vi "Tap Handler.vi"(8 "error in (no error)":errorcluster) -> (0 "error out":errorcluster)   [LabVIEW 2014]
uses:
  STD - Tap Mode.ctl
  Globals.vi
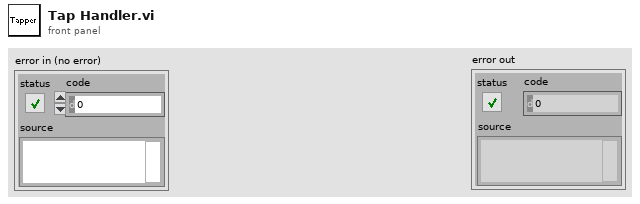
[diagram p1: front panel]
types:
  T1 = typedef "STD - Tap Mode.ctl" = enum32{"No Action", "Stay Level", "Rise", "Fall", "Calibrate"}
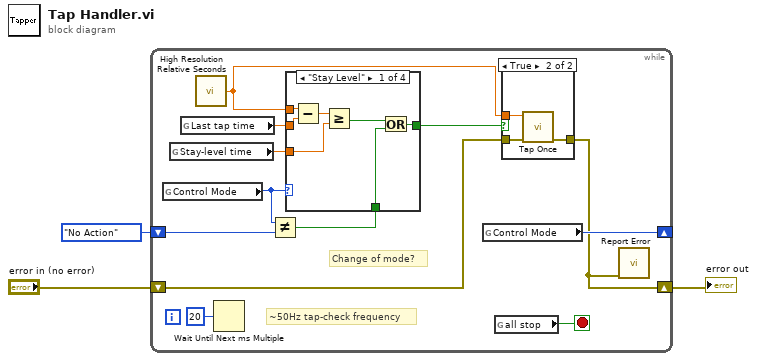
[diagram p0: block diagram]
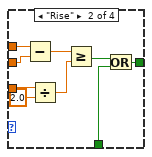
[diagram p2: hidden frame]
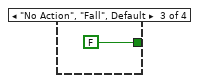
[diagram p3: hidden frame]
diagram:
  n1 = while {
    shift-right: [w11] -> _
    shift-left: STD_-_Tap_Mode."No Action" ("Control Mode") -> [w10]
    shift-right: [w4] -> w2
    shift-left: "error in (no error)" -> [w6]
    stop <- w7 stop-if-true
    # "Change of mode?"
    # "~50Hz tap-check frequency"
    n2 = global read "Globals.vi" "Control Mode"() -> (w12:T1)
    n3 = global read "Globals.vi" "Stay-level time"() -> (w13:dbl)
    n4 = global read "Globals.vi" "Last tap time"() -> (w14:dbl)
    n5 = call <vilib>:"High Resolution Relative Seconds.vi"() -> ("relative seconds"=w5:dbl)
    n6 = Wait Until Next ms Multiple(millisecond multiple=u32 20) -> ()  [unwired: 1 out]
    n7 = Not Equal?(x=w12, y=w10) -> (x != y?=w8:bool)
    n8 = case shown="\"Stay Level\"" w12 {
      tunnel: [w19 w26 FALSE w33] -> w9
      tunnel: w14 -> [w22 w29 _ _]
      tunnel: w13 -> [w20 w31 _ _]
      tunnel: w8 -> [w17 w24 _ w33]
      tunnel: w5 -> [w16 w23 _ _]
      frame "Stay Level" {
        n9 = Subtract(x=w16, y=w22) -> (x-y=w21:dbl)
        n10 = Greater Or Equal?(x=w21, y=w20) -> (x >= y?=w18:bool)
        n11 = Or(x=w18, y=w17) -> (x .or. y?=w19:bool)
      }
      frame "Rise" {
        n12 = Subtract(x=w23, y=w29) -> (x-y=w28:dbl)
        n13 = Divide(x=w31, y=2.0) -> (x/y=w27:dbl)
        n14 = Greater Or Equal?(x=w28, y=w27) -> (x >= y?=w25:bool)
        n15 = Or(x=w25, y=w24) -> (x .or. y?=w26:bool)
      }
      frame "No Action", "Fall", Default {
      }
      frame "Calibrate" {
      }
    }
    n16 = global read "Globals.vi" "Control Mode"() -> (w11:T1)
    n17 = global read "Globals.vi" "all stop"() -> (w7:bool)
    n18 = case shown="True" w9 {
      tunnel: w6 -> [w34 w37]
      tunnel: [w34 w36] -> w4
      tunnel: w5 -> [_ w35]
      frame False {
      }
      frame True {
        n19 = call "Tap Once.vi"("error in (no error)"=w37, "Call time (s)"=w35) -> ("error out"=w36:errorcluster)  [unwired: 9 in]
      }
    }
    n20 = call "Report Error.vi"("error in (no error)"=w4) -> ()  [unwired: 11 in]
  }
  "error out" <- w2
